vi "aal_DZT.vi"   [LabVIEW 2020, in "NI_AALPro.lvlib"]
uses:
  NI_AALPro.lvlib
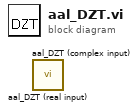
[diagram p0: block diagram]
diagram:
  n1 = call "aal_DZT (real input).vi"() -> ()  [unwired: 5 in, 2 out]
  n2 = call "aal_DZT (complex input).vi"() -> ()  [unwired: 5 in, 2 out]
